vi "Filter.vi"(8 "Ts (s)":dbl=0.1, 9 "Filter Level":dbl, 11 "Input":dbl) -> (3 "Output":dbl)   [LabVIEW 2020, in "Common.lvlib"]
uses:
  Common.lvlib
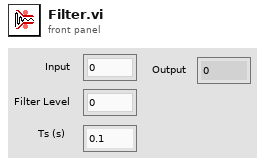
[diagram p1: front panel]
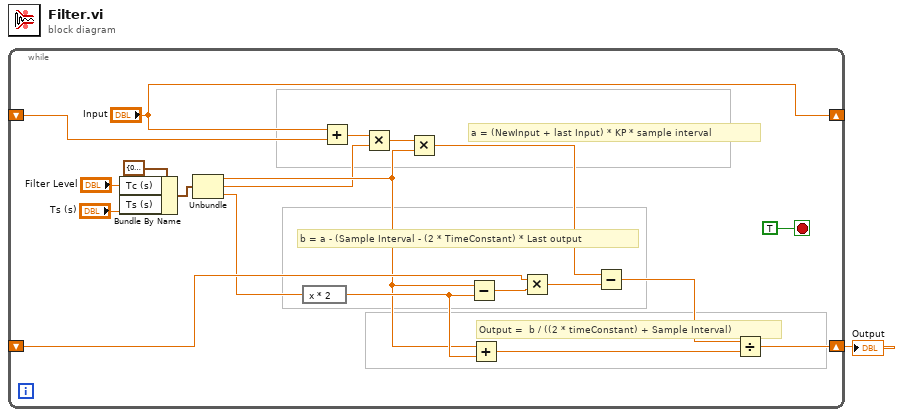
[diagram p0: block diagram]
diagram:
  n1 = while {
    shift-right: ["Input"] -> _
    shift-left: _ -> [w20]
    shift-right: [w21] -> w1
    shift-left: _ -> [w18]
    stop <- TRUE stop-if-true
    # "Output =  b / ((2 * timeConstant) + Sample Interval)"
    # "b = a - (Sample Interval - (2 * TimeConstant) * Last output"
    # "a = (NewInput + last Input) * KP * sample interval"
    n2 = Bundle By Name(cluster=cluster{" Ts (s)":dbl, "Gain":dbl, "Tc (s)":dbl} {" Ts (s)"=0.1, "Gain"=1.0, "Tc (s)"=20.0} ("Parameters"), "Tc (s)"="Filter Level", "Ts (s)"="Ts (s)") -> (w4:cluster{" Ts (s)":dbl, "Gain":dbl, "Tc (s)":dbl})
    n3 = Unbundle(w4) -> ("Ts (s)"=w12:dbl, "Gain"=w11:dbl, "Tc (s)"=w10:dbl)
    n4 = expression code="x * 2"(w10) -> (w14:dbl)
    n5 = Add(x="Input", y=w20) -> (x+y=w17:dbl)
    n6 = Multiply(x=w17, y=w11) -> (x*y=w16:dbl)
    n7 = Multiply(x=w16, y=w12) -> (x*y=w7:dbl)
    n8 = Subtract(x=w12, y=w14) -> (x-y=w15:dbl)
    n9 = Add(x=w12, y=w14) -> (x+y=w13:dbl)
    n10 = Multiply(x=w18, y=w15) -> (x*y=w9:dbl)
    n11 = Subtract(x=w7, y=w9) -> (x-y=w8:dbl)
    n12 = Divide(x=w8, y=w13) -> (x/y=w21:dbl)
  }
  "Output" <- w1
